vi "Calculul FFT unilaterala.vi"() -> ()   [LabVIEW 2011]
uses:
  <vilib>/Analysis/2dsp.llb/Real FFT.vi
  <vilib>/Analysis/NI_AALBase.lvlib
  <vilib>/Analysis/NI_AALPro.lvlib
panel:
  out "Spectrul":cluster{i32, dbl, dbl[]}(graph)
  out "semnalul in domeniul timp":dbl[](graph)
  in  "Amplitudinea":dbl
  in  "nr de esantionare":i32
  in  "frecventa de esantionare [Hz]":dbl
  in  "frecventa [Hz]":dbl
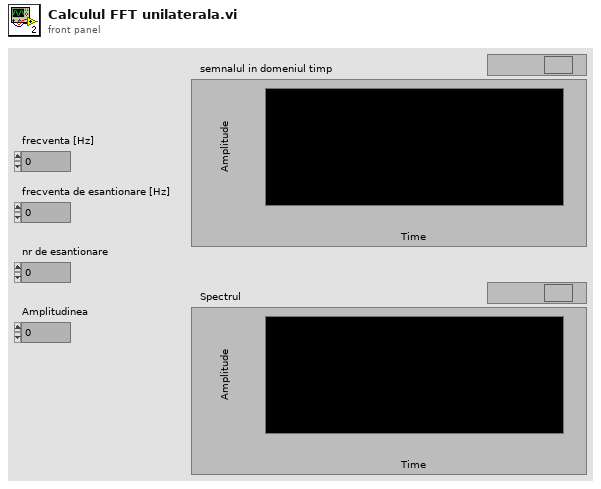
[diagram p1: front panel]
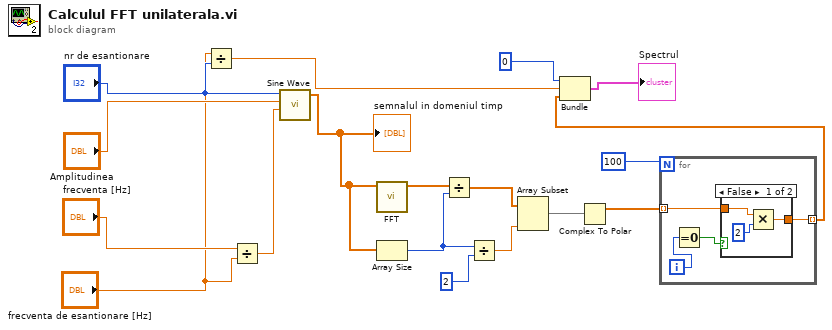
[diagram p0: block diagram]
diagram:
  n1 = Divide(x="frecventa de esantionare [Hz]", y="nr de esantionare") -> (x/y=w14:dbl)
  n2 = Divide(x="frecventa [Hz]", y="frecventa de esantionare [Hz]") -> (x/y=w1:dbl)
  n3 = call <vilib>:"Sine Wave.vi"("samples"="nr de esantionare", "amplitude"="Amplitudinea", "frequency"=w1) -> ("sine wave"=w13:dbl[])  [unwired: 2 in, 2 out]
  "semnalul in domeniul timp" <- w13
  n4 = call-poly <vilib>:"FFT.vi"("X"=w13) -> ("FFT {X}"=w12:cdb[])  [unwired: 9 in, 1 out]
  n5 = Array Size(array=w13) -> (size(s)=w10:i32)
  n6 = Divide(x=w12, y=w10) -> (x/y=w8:cdb[])
  n7 = Divide(x=w10, y=2) -> (x/y=w9:dbl)
  n8 = Array Subset(array=w8, length=w9) -> (w7:cdb[])  [unwired: 1 in]
  n9 = Complex To Polar(r * e^(i*theta)=w7) -> (r=w18:dbl[])  [unwired: 1 out]
  n10 = for {
    N: 100 -> [_]
    tunnel: [w22] -> w17 mode=indexing
    tunnel: w18 -> [w19] mode=indexing
    i -> [w20]
    n11 = Equal To 0?(x=w20) -> (x = 0?=w21:bool)
    n12 = case shown="False" w21 {
      tunnel: [w24 w26] -> w22
      tunnel: w19 -> [w23 w26]
      frame False {
        n13 = Multiply(x=w23, y=2) -> (x*y=w24:dbl)
      }
      frame True {
      }
    }
  }
  n14 = Bundle(0, w14, w17) -> (→"Spectrul":cluster{i32, dbl, dbl[]})  [unwired: 1 in]
